vi "UpdateApprovedHawkList.vi"(8 "error in (no error)":errorcluster, 10 "ApprovedDeps Cluster":T1, 11 "Config Refnum in":T2) -> (0 "error out":errorcluster, 3 "Config Refnum out":T2)   [LabVIEW 2019, in "Hawkeye.lvlib"]
uses:
  Hawkeye.lvlib
  <vilib>/Utility/config.llb/Config Data RefNum.ctl
  Typedefs/ConfirmDeps.ctl
  <vilib>/Utility/config.llb/Write Key (String).vi
  <vilib>/Utility/config.llb/NI_LVConfig.lvlib
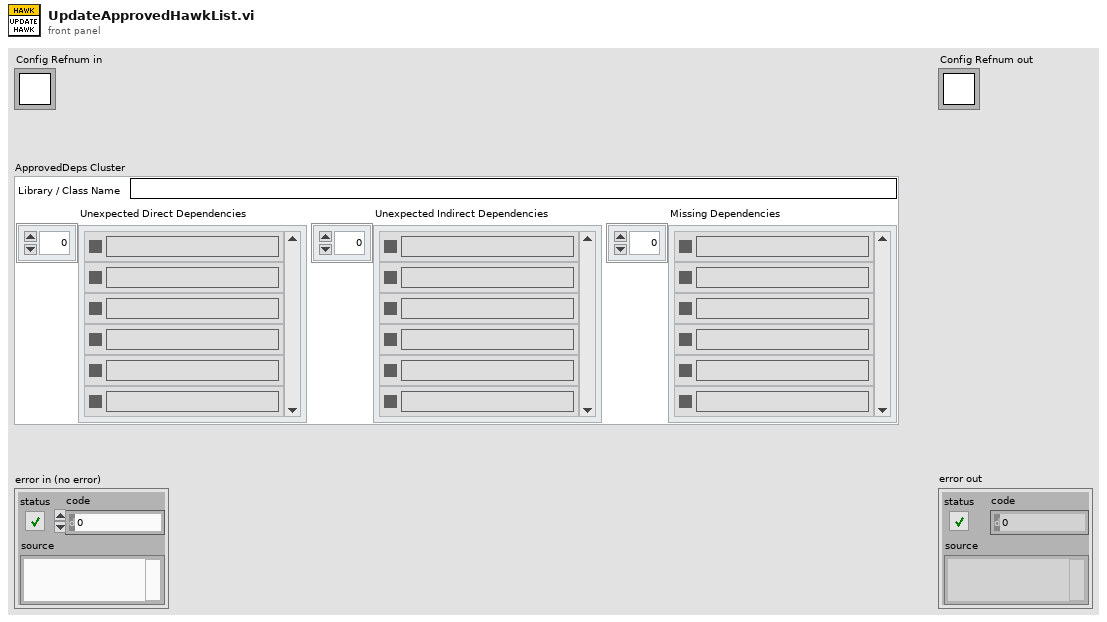
[diagram p1: front panel]
types:
  T1 = typedef "Hawkeye.lvlib/ConfirmDeps.ctl" = cluster{"Library / Class Name":string, "Unexpected Direct Dependencies":cluster{"Confirm Status":enum8{"False", "True", "Mixed"}, "Library / Class Name":string}[], "Unexpected Indirect Dependencies":cluster{"Confirm Status":enum8{"False", "True", "Mixed"}, "Library / Class Name":string}[], "Missing Dependencies":cluster{"Confirm Status":enum8{"False", "True", "Mixed"}, "Library / Class Name":string}[]}
  T2 = typedef "NI_LVConfig.lvlib/Config Data RefNum.ctl" = refnum<k1>
  T3 = cluster{"Confirm Status":enum8{"False", "True", "Mixed"}, "Library / Class Name":string}[]
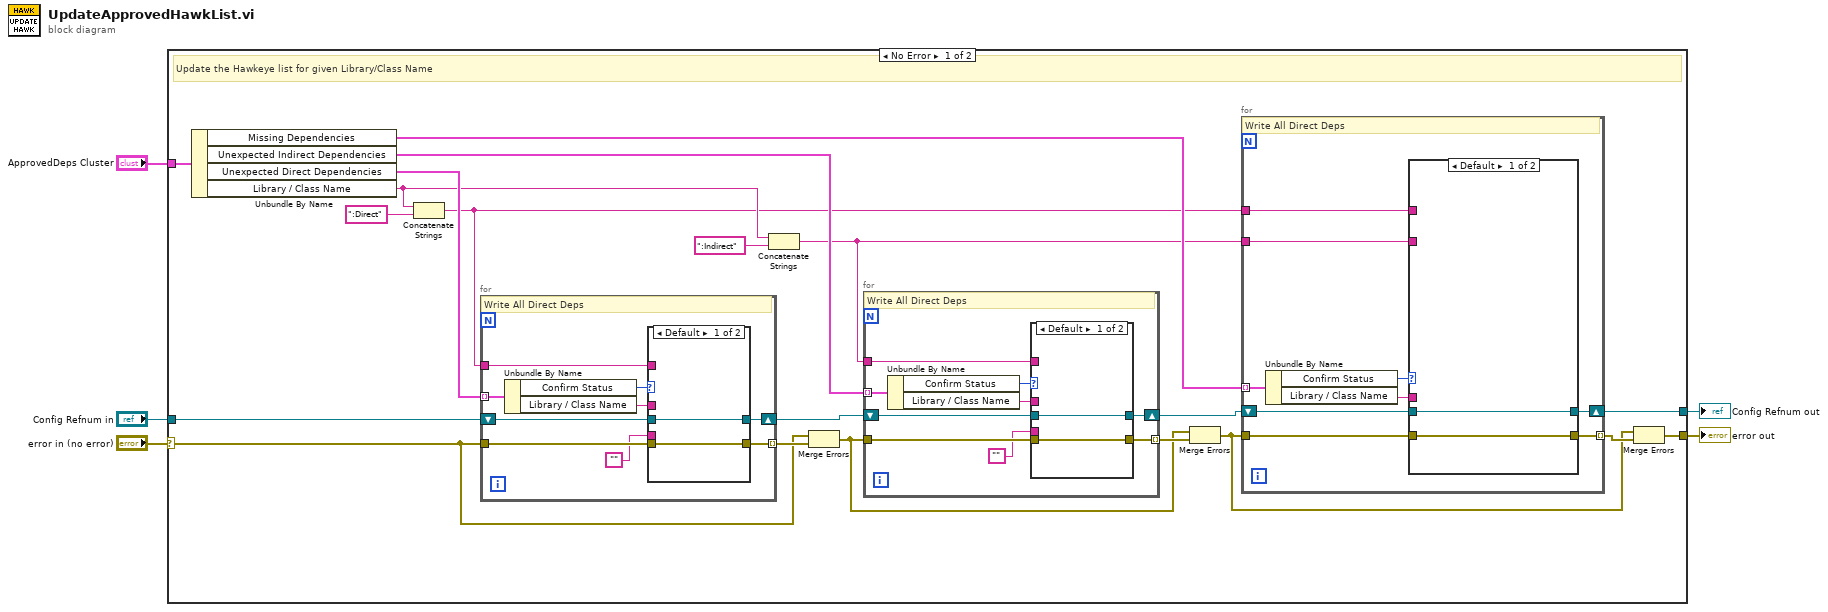
[diagram p0: block diagram]
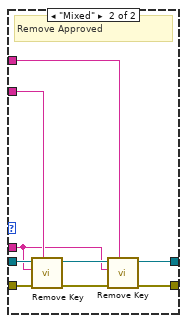
[diagram p2: hidden frame]
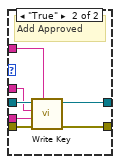
[diagram p3: hidden frame]
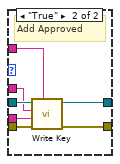
[diagram p4: hidden frame]
diagram:
  n1 = case shown="No Error" "error in (no error)" {
    selector: "error in (no error)" -> [w19 w83]
    tunnel: "Config Refnum in" -> [w23 w82]
    tunnel: [w10 w82] -> w4
    tunnel: [w21 w83] -> w2
    tunnel: "ApprovedDeps Cluster" -> [w20 _]
    frame No Error {
      # "Update the Hawkeye list for given Library/Class Name"
      n2 = Unbundle By Name(w20) -> ("Missing Dependencies"=w14:T3, "Unexpected Indirect Dependencies"=w17:T3, "Unexpected Direct Dependencies"=w18:T3, "Library / Class Name"=w15:string)
      n3 = Concatenate Strings(w15, ":Direct" ("Type")) -> (w9:string)
      n4 = for {
        tunnel: w9 -> [w72]
        shift-right: [w70] -> w16
        shift-left: w23 -> [w71]
        tunnel: w19 -> [w69]
        tunnel: [w68] -> w22 mode=indexing
        tunnel: w18 -> [w66] mode=indexing
        # "Write All Direct Deps"
        n5 = Unbundle By Name(w66) -> ("Confirm Status"=w64:enum8{"False", "True", "Mixed"}, "Library / Class Name"=w65:string)
        n6 = case shown="Default" w64 {
          tunnel: w72 -> [_ w81]
          tunnel: w71 -> [w74 w80]
          tunnel: [w74 w79] -> w70
          tunnel: w69 -> [w73 w78]
          tunnel: [w73 w77] -> w68
          tunnel: "" -> [_ w76]
          tunnel: w65 -> [_ w75]
          frame Default {
          }
          frame "True" {
            # "Add Approved"
            n7 = call-poly <vilib>:"Write Key.vi"("section"=w81, "error in (no error)"=w78, "value"=w76, "key"=w75, "refnum"=w80) -> ("error out"=w77:errorcluster, "refnum out"=w79:T2)  [unwired: 4 in, 1 out]
          }
        }
      }
      n8 = Concatenate Strings(w15, ":Indirect" ("Type")) -> (w8:string)
      n9 = Merge Errors(w19, w22) -> (w7:errorcluster)
      n10 = for {
        tunnel: w8 -> [w54]
        shift-right: [w52] -> w12
        shift-left: w16 -> [w53]
        tunnel: w7 -> [w51]
        tunnel: [w50] -> w13 mode=indexing
        tunnel: w17 -> [w48] mode=indexing
        # "Write All Direct Deps"
        n11 = Unbundle By Name(w48) -> ("Confirm Status"=w46:enum8{"False", "True", "Mixed"}, "Library / Class Name"=w47:string)
        n12 = case shown="Default" w46 {
          tunnel: w54 -> [_ w63]
          tunnel: w53 -> [w56 w62]
          tunnel: [w56 w61] -> w52
          tunnel: w51 -> [w55 w60]
          tunnel: [w55 w59] -> w50
          tunnel: "" -> [_ w58]
          tunnel: w47 -> [_ w57]
          frame Default {
          }
          frame "True" {
            # "Add Approved"
            n13 = call-poly <vilib>:"Write Key.vi"("section"=w63, "error in (no error)"=w60, "value"=w58, "key"=w57, "refnum"=w62) -> ("error out"=w59:errorcluster, "refnum out"=w61:T2)  [unwired: 4 in, 1 out]
          }
        }
      }
      n14 = Merge Errors(w7, w13) -> (w6:errorcluster)
      n15 = for {
        tunnel: w9 -> [w34]
        shift-right: [w32] -> w10
        shift-left: w12 -> [w33]
        tunnel: w6 -> [w31]
        tunnel: [w30] -> w11 mode=indexing
        tunnel: w14 -> [w29] mode=indexing
        tunnel: w8 -> [w26]
        # "Write All Direct Deps"
        n16 = Unbundle By Name(w29) -> ("Confirm Status"=w27:enum8{"False", "True", "Mixed"}, "Library / Class Name"=w28:string)
        n17 = case shown="Default" w27 {
          tunnel: w34 -> [_ w38]
          tunnel: w33 -> [w36 w45]
          tunnel: [w36 w42] -> w32
          tunnel: w31 -> [w35 w44]
          tunnel: [w35 w41] -> w30
          tunnel: w28 -> [_ w37]
          tunnel: w26 -> [_ w39]
          frame Default {
          }
          frame "Mixed" {
            # "Remove Approved"
            n18 = call <vilib>:"Remove Key.vi"("section"=w39, "error in (no error)"=w44, "key"=w37, "refnum"=w45) -> ("error out"=w40:errorcluster, "refnum out"=w43:T2)  [unwired: 5 in, 1 out]
            n19 = call <vilib>:"Remove Key.vi"("section"=w38, "error in (no error)"=w40, "key"=w37, "refnum"=w43) -> ("error out"=w41:errorcluster, "refnum out"=w42:T2)  [unwired: 5 in, 1 out]
          }
        }
      }
      n20 = Merge Errors(w6, w11) -> (w21:errorcluster)
    }
    frame Error {
    }
  }
  "error out" <- w2
  "Config Refnum out" <- w4
